vi "Find Gaps on Particular Machine.vi"(9 "Number of Scheduled Jobs on This Machine":i32, 11 "Gannt Chart For Machine In":T2[](array[typedef])) -> (2 "Gaps":T1[](array[typedef]))   [LabVIEW 2013, in "GanntChart.lvclass"]
uses:
  GanntChart.lvclass
  Controls/GanntChart_Element.ctl
  Controls/Gap.ctl
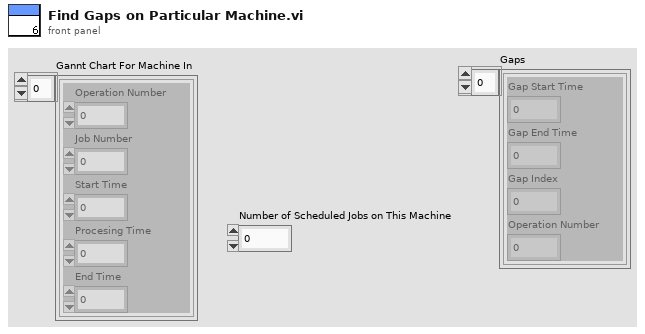
[diagram p1: front panel]
types:
  T1 = typedef "Gap.ctl" = cluster{"Gap Start Time":i32, "Gap End Time":i32, "Gap Index":i32, "Operation Number":i32}
  T2 = typedef "GanntChart_Element.ctl" = cluster{"Operation Number":i32, "Job Number":i32, "Start Time":i32, "Procesing Time":u16, "End Time":i32}
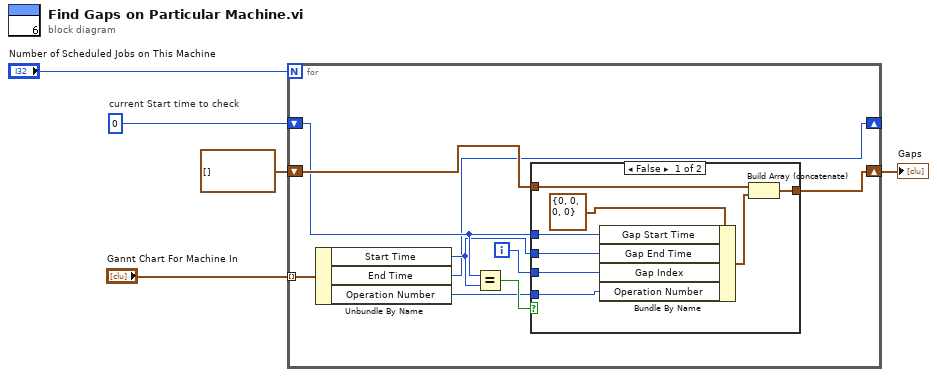
[diagram p0: block diagram]
diagram:
  w4 = 0  # current Start time to check
  n1 = for {
    N: "Number of Scheduled Jobs on This Machine" -> [_]
    tunnel: "Gannt Chart For Machine In" -> [w14] mode=indexing
    shift-right: [w8] -> _
    shift-left: w4 -> [w11]
    shift-right: [w9] -> w2
    shift-left: T1[] [] -> [w12]
    i -> [w7]
    n2 = Unbundle By Name(w14) -> ("Start Time"=w10:i32, "End Time"=w8:i32, "Operation Number"=w6:i32)
    n3 = Equal?(x=w11, y=w10) -> (x = y?=w13:bool)
    n4 = case shown="False" w13 {
      tunnel: w12 -> [w19 w23]
      tunnel: w11 -> [w21 _]
      tunnel: w10 -> [w20 _]
      tunnel: [w17 w23] -> w9
      tunnel: w7 -> [w16 _]
      tunnel: w6 -> [w15 _]
      frame False {
        n5 = Bundle By Name(cluster=T1 {"Gap Start Time"=0, "Gap End Time"=0, "Gap Index"=0, "Operation Number"=0}, "Gap Start Time"=w21, "Gap End Time"=w20, "Gap Index"=w16, "Operation Number"=w15) -> (w18:T1)
        n6 = Build Array (concatenate)(w19, w18) -> (w17:T1[])
      }
      frame True {
      }
    }
  }
  "Gaps" <- w2
